vi "Write output H.vi"(10 "output H":dbl=100.0 format="%.2f", 11 "Impulsator in":refnum<class "Impulsator.lvclass">) -> (3 "Impulsator out":refnum<class "Impulsator.lvclass">)   [LabVIEW 2019, in "Userlib.lvlib" / "Impulsator.lvclass"]
uses:
  Impulsator.lvclass
  Impulsator.lvclass/Impulsator.ctl
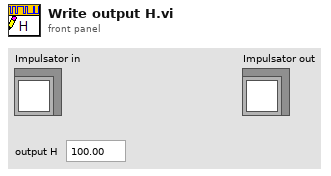
[diagram p1: front panel]
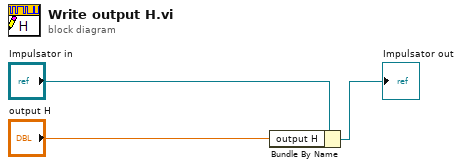
[diagram p0: block diagram]
diagram:
  n1 = Bundle By Name(cluster="Impulsator in", "output H"="output H") -> (→"Impulsator out":refnum<class "Impulsator.lvclass">)
